vi "FPDAQtoDAQstrings.vi"(1 "front panel":T1={"AO Configuration"=[], "AI Configuration"=[], "Channels: AO"=[], "Channels: Lockin"=[{"Enable?"=FALSE, "Channel"=13, "Frequency"=0.1, "Phase"=0.0, "TC"=1e-05, "Roll-Off"=1}], "DAQ Type"=enum."None", "Amplifiers"=enum."Manual", "Gain"=[], "offsets"=[], "Cal Info"=[], "TC (s)"=0.0, "order"=0, "60 Hz prefilter"=FALSE, "LP prefilter"=FALSE, "LP cutoff (Hz)"=0.0, "Fs"=0, "#s"=0} {"AI Configuration"."AI.Coupling" items=["AC"=10045, "DC"=10050, "GND"=10066]; "Channels: AO"."Phase" format="%.3g"; "Channels: AO"."Frequency" min=0.0001 max=10000.0 format="%.3g"; "Channels: AO"."Offset" format="%.3p"; "Channels: AO"."Amplitude" min=0.0 max=10.0 format="%.3p"; "Channels: Lockin"."Roll-Off" min=1; "Channels: Lockin"."TC" min=0.0001 format="%#_3p"; "Channels: Lockin"."Phase" format="%.3g"; "Channels: Lockin"."Frequency" min=0.0001 max=10000.0 format="%.3g"; "Cal Info"."SelfCal.LastDate/Time" format="%<%I:%M %p\n%m/%d/%Y>T"}) -> (0 "front panel (DAQmx strings)":T17={"AO Configuration"=[], "AI Configuration"=[], "Channels: AO"=[], "Channels: Lockin"=[{"Enable?"=FALSE, "Channel"=13, "Frequency"=0.1, "Phase"=0.0, "TC"=1e-05, "Roll-Off"=1}], "DAQ Type"=enum."None", "Amplifiers"=enum."Manual", "Gain"=[], "offsets"=[], "Cal Info"=[], "TC (s)"=0.0, "order"=0, "60 Hz prefilter"=FALSE, "LP prefilter"=FALSE, "LP cutoff (Hz)"=0.0, "Fs"=0, "#s"=0} {"AI Configuration"."AI.Coupling" items=["AC"=10045, "DC"=10050, "GND"=10066]; "Channels: AO"."Phase" format="%.3g"; "Channels: AO"."Frequency" min=0.0001 max=10000.0 format="%.3g"; "Channels: AO"."Offset" format="%.3p"; "Channels: AO"."Amplitude" min=0.0 max=10.0 format="%.3p"; "Channels: Lockin"."Roll-Off" min=1; "Channels: Lockin"."TC" min=0.0001 format="%#_3p"; "Channels: Lockin"."Phase" format="%.3g"; "Channels: Lockin"."Frequency" min=0.0001 max=10000.0 format="%.3g"})   [LabVIEW 2019, in "Instrument.DAQ.lvclass"]
uses:
  Instrument.DAQ.lvclass
  Typedefs/446xAO-enum.ctl
  Typedefs/446xAI-enum.ctl
  Typedefs/AI.coupling-enum.ctl
  Typedefs/AmplifierType-enum.ctl
  Typedefs/DAQType-enum.ctl
  Typedefs/REF-cluster.ctl
  Typedefs/Function-enum.ctl
  Typedefs/AO-cluster.ctl
  Instrument UI.Lockin/Typedefs/REF Channel--Cluster.ctl
  Instrument UI.Lockin/Instrument UI.Lockin.lvclass
  Instrument UI.Lockin/Typedefs/AO Channel--Cluster.ctl
  Typedefs/Cal Info - Cluster.ctl
  Typedefs/AI.config(UI)-cluster.ctl
  Typedefs/AI.config(UI)-array.ctl
  Typedefs/AO.config(UI)-cluster.ctl
  Typedefs/AO.config(UI)-array.ctl
  Typedefs/Front Panel Cluster.ctl
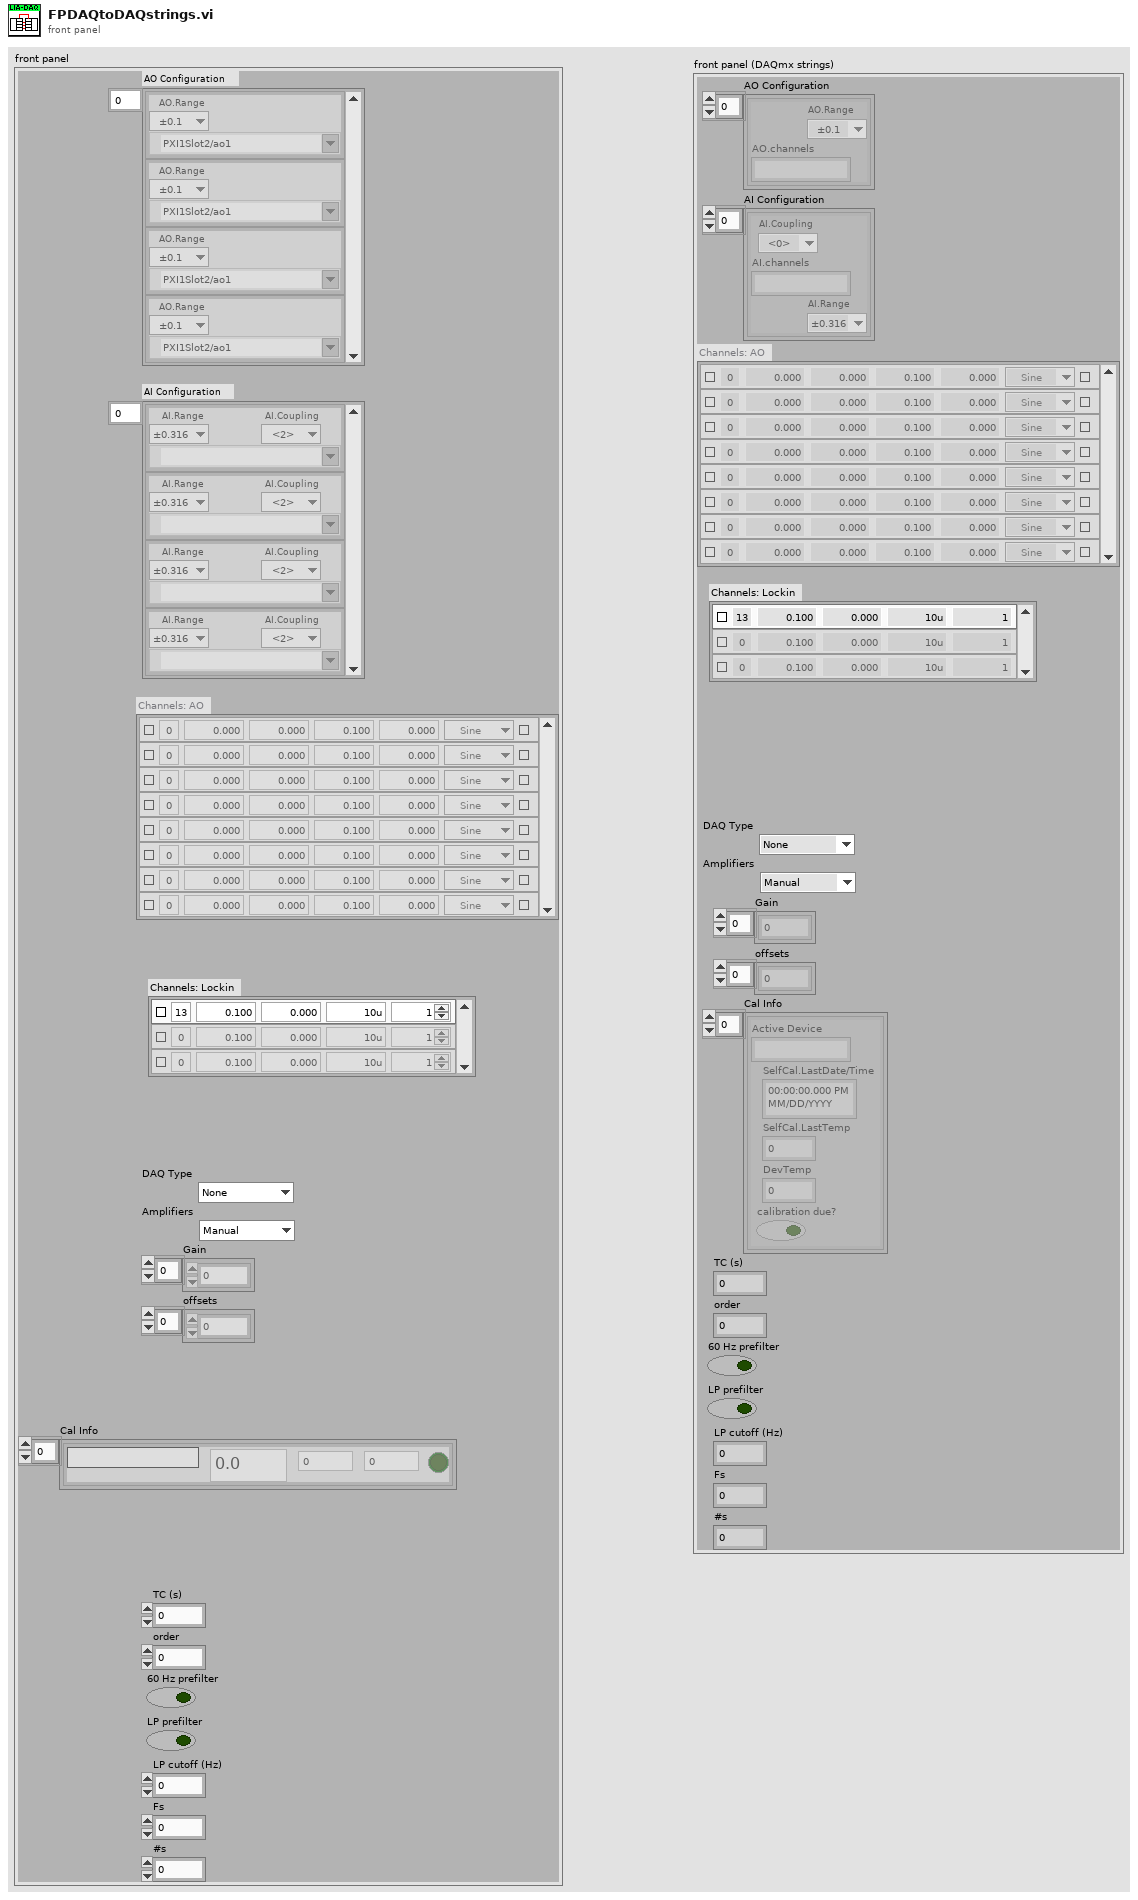
[diagram p1: front panel]
types:
  T1 = typedef "Instrument.DAQ.lvclass/Front Panel Cluster.ctl" = cluster{"AO Configuration":T2, "AI Configuration":T5, "Channels: AO":T9, "Channels: Lockin":T12, "DAQ Type":T14, "Amplifiers":T15, "Gain":dbl[], "offsets":dbl[], "Cal Info":T16[], "TC (s)":dbl, "order":i32, "60 Hz prefilter":bool, "LP prefilter":bool, "LP cutoff (Hz)":dbl, "Fs":i32, "#s":i32}
  T2 = typedef "Instrument.DAQ.lvclass/AO.config(UI)-array.ctl" = T3[]
  T3 = typedef "Instrument.DAQ.lvclass/AO.config(UI)-cluster.ctl" = cluster{"AO.Range":T4, "AO.channels":tag}
  T4 = typedef "Instrument.DAQ.lvclass/446xAO-enum.ctl" = enum16{"±0.1", "±1.0", "±10.0"}
  T5 = typedef "Instrument.DAQ.lvclass/AI.config(UI)-array.ctl" = T6[]
  T6 = typedef "Instrument.DAQ.lvclass/AI.config(UI)-cluster.ctl" = cluster{"AI.Coupling":T7, "AI.channels":tag, "AI.Range":T8}
  T7 = typedef "Instrument.DAQ.lvclass/AI.coupling-enum.ctl" = u16
  T8 = typedef "Instrument.DAQ.lvclass/446xAI-enum.ctl" = enum16{"±0.316", "±1.00", "±3.16", "±10.0", "±31.6", "±42.4"}
  T9 = typedef "Instrument.DAQ.lvclass/AO-cluster.ctl" = T10[]
  T10 = typedef "Instrument UI.Lockin.lvclass/AO Channel--Cluster.ctl" = cluster{"Enable?":bool, "Channel":i32, "Amplitude":dbl, "Offset":dbl, "Frequency":dbl, "Phase":dbl, "Function":T11, "Sweeping?":bool}
  T11 = typedef "Instrument.DAQ.lvclass/Function-enum.ctl" = enum16{"Sine", "Triangle", "Square"}
  T12 = typedef "Instrument.DAQ.lvclass/REF-cluster.ctl" = T13[]
  T13 = typedef "Instrument UI.Lockin.lvclass/REF Channel--Cluster.ctl" = cluster{"Enable?":bool, "Channel":i32, "Frequency":dbl, "Phase":dbl, "TC":dbl, "Roll-Off":i32}
  T14 = typedef "Instrument.DAQ.lvclass/DAQType-enum.ctl" = enum16{"None", "USB 4431", "PXI 446x"}
  T15 = typedef "Instrument.DAQ.lvclass/AmplifierType-enum.ctl" = enum16{"Manual", "Krohn Hite", "Femto"}
  T16 = typedef "Instrument.DAQ.lvclass/Cal Info - Cluster.ctl" = cluster{"Active Device":string, "SelfCal.LastDate/Time":dbl, "SelfCal.LastTemp":dbl, "DevTemp":dbl, "calibration due?":bool}
  T17 = cluster{"AO Configuration":cluster{"AO.Range":T4, "AO.channels":string}[], "AI Configuration":cluster{"AI.Coupling":T7, "AI.channels":string, "AI.Range":T8}[], "Channels: AO":T9, "Channels: Lockin":T12, "DAQ Type":T14, "Amplifiers":T15, "Gain":dbl[], "offsets":dbl[], "Cal Info":cluster{"Active Device":string, "SelfCal.LastDate/Time":timestamp, "SelfCal.LastTemp":dbl, "DevTemp":dbl, "calibration due?":bool}[], "TC (s)":dbl, "order":i32, "60 Hz prefilter":bool, "LP prefilter":bool, "LP cutoff (Hz)":dbl, "Fs":i32, "#s":i32}
  T18 = cluster{"AI.Coupling":T7, "AI.channels":string, "AI.Range":T8}
  T19 = cluster{"Active Device":string, "SelfCal.LastDate/Time":timestamp, "SelfCal.LastTemp":dbl, "DevTemp":dbl, "calibration due?":bool}
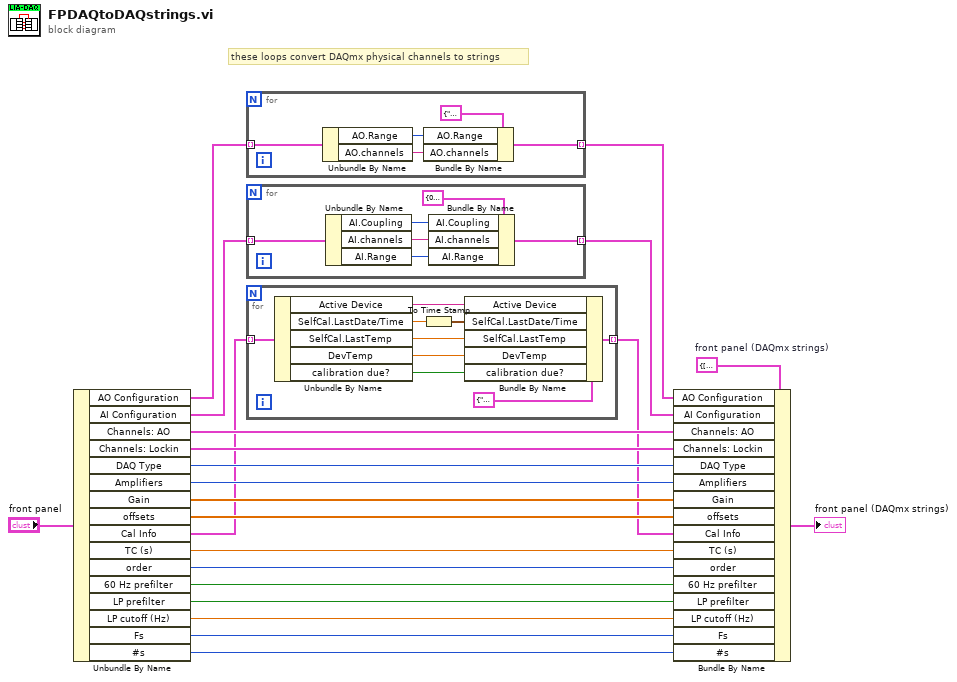
[diagram p0: block diagram]
diagram:
  w22 = T17 {"AO Configuration"=[], "AI Configuration"=[], "Channels: AO"=[], "Channels: Lockin"=[{"Enable?"=FALSE, "Channel"=13, "Frequency"=0.1, "Phase"=0.0, "TC"=1e-05, "Roll-Off"=1}], "DAQ Type"=enum."None", "Amplifiers"=enum."Manual", "Gain"=[], "offsets"=[], "Cal Info"=[], "TC (s)"=0.0, "order"=0, "60 Hz prefilter"=FALSE, "LP prefilter"=FALSE, "LP cutoff (Hz)"=0.0, "Fs"=0, "#s"=0}  # front panel (DAQmx strings)
  # "these loops convert DAQmx physical channels to strings"
  n1 = Unbundle By Name("front panel") -> ("AO Configuration"=w20:T2, "AI Configuration"=w19:T5, "Channels: AO"=w18:T9, "Channels: Lockin"=w17:T12, "DAQ Type"=w16:T14, "Amplifiers"=w15:T15, "Gain"=w14:dbl[], "offsets"=w13:dbl[], "Cal Info"=w12:T16[], "TC (s)"=w11:dbl, "order"=w10:i32, "60 Hz prefilter"=w9:bool, "LP prefilter"=w8:bool, "LP cutoff (Hz)"=w7:dbl, "Fs"=w6:i32, "#s"=w5:i32)
  n2 = for {
    tunnel: w20 -> [w27] mode=indexing
    tunnel: [w25] -> w2 mode=indexing
    n3 = Unbundle By Name(w27) -> ("AO.Range"=w26:T4, "AO.channels"=w23:tag)
    n4 = Bundle By Name(cluster=cluster{"AO.Range":T4, "AO.channels":string} {"AO.Range"=enum."±0.1", "AO.channels"=""}, "AO.Range"=w26, "AO.channels"=w23) -> (w25:cluster{"AO.Range":T4, "AO.channels":string})
  }
  n5 = for {
    tunnel: w19 -> [w33] mode=indexing
    tunnel: [w32] -> w3 mode=indexing
    n6 = Unbundle By Name(w33) -> ("AI.Coupling"=w28:T7, "AI.channels"=w29:tag, "AI.Range"=w30:T8)
    n7 = Bundle By Name(cluster=T18 {"AI.Coupling"=0, "AI.channels"="", "AI.Range"=enum."±0.316"}, "AI.Coupling"=w28, "AI.channels"=w29, "AI.Range"=w30) -> (w32:T18)
  }
  n8 = for {
    tunnel: w12 -> [w41] mode=indexing
    tunnel: [w42] -> w4 mode=indexing
    n9 = Unbundle By Name(w41) -> ("Active Device"=w35:string, "SelfCal.LastDate/Time"=w36:dbl, "SelfCal.LastTemp"=w37:dbl, "DevTemp"=w38:dbl, "calibration due?"=w39:bool)
    n10 = To Time Stamp(1:w36) -> (0:w34:timestamp)
    n11 = Bundle By Name(cluster=T19 {"Active Device"="", "SelfCal.LastDate/Time"=timestamp(0 s since 1904-01-01), "SelfCal.LastTemp"=0.0, "DevTemp"=0.0, "calibration due?"=FALSE}, "Active Device"=w35, "SelfCal.LastDate/Time"=w34, "SelfCal.LastTemp"=w37, "DevTemp"=w38, "calibration due?"=w39) -> (w42:T19)
  }
  n12 = Bundle By Name(cluster=w22, "AO Configuration"=w2, "AI Configuration"=w3, "Channels: AO"=w18, "Channels: Lockin"=w17, "DAQ Type"=w16, "Amplifiers"=w15, "Gain"=w14, "offsets"=w13, "Cal Info"=w4, "TC (s)"=w11, "order"=w10, "60 Hz prefilter"=w9, "LP prefilter"=w8, "LP cutoff (Hz)"=w7, "Fs"=w6, "#s"=w5) -> (→"front panel (DAQmx strings)":T17)
